vi "3.7.4-UDP-Forbrain_to_OCU-Server.vi"() -> ()   [LabVIEW 2010]
doc: "Creates a named service and listens on the first available port. Whenever a client connects to the service, it responds with a message containing joystick data. The VI can be stopped using the STOP button."
uses:
  6-OCU Neurons/CommonIndicators.ctl
  5.0-Global.vi
panel:
  out "5.7.2 Main Indicators":T1={"Speed"=0.0, " Heading"={0.0, 34.390870865624734}, "MissionTime"=0.0, "Battery"=0.0, "MAP"=FALSE, "LIDAR"=FALSE, "ManualMissionMap"=bytes[0], "ManualModeLIDAR"=bytes[0], "ManualModeStop"=FALSE, "How? 2"=FALSE, "Where? 2"=FALSE, "MWhat?"=FALSE, "ActManual"=FALSE, "CollisionLight"=FALSE, "CollisionLight 2"=FALSE, "Ready"=FALSE} {"Battery" scale=16.0..24.0; "MissionTime" scale=0.0..10.0; "Heading" scale=180.0..-180.0; "Speed" scale=0.0..4.0}
  out "data out":string
  out "error out":errorcluster
  in  "error in":errorcluster
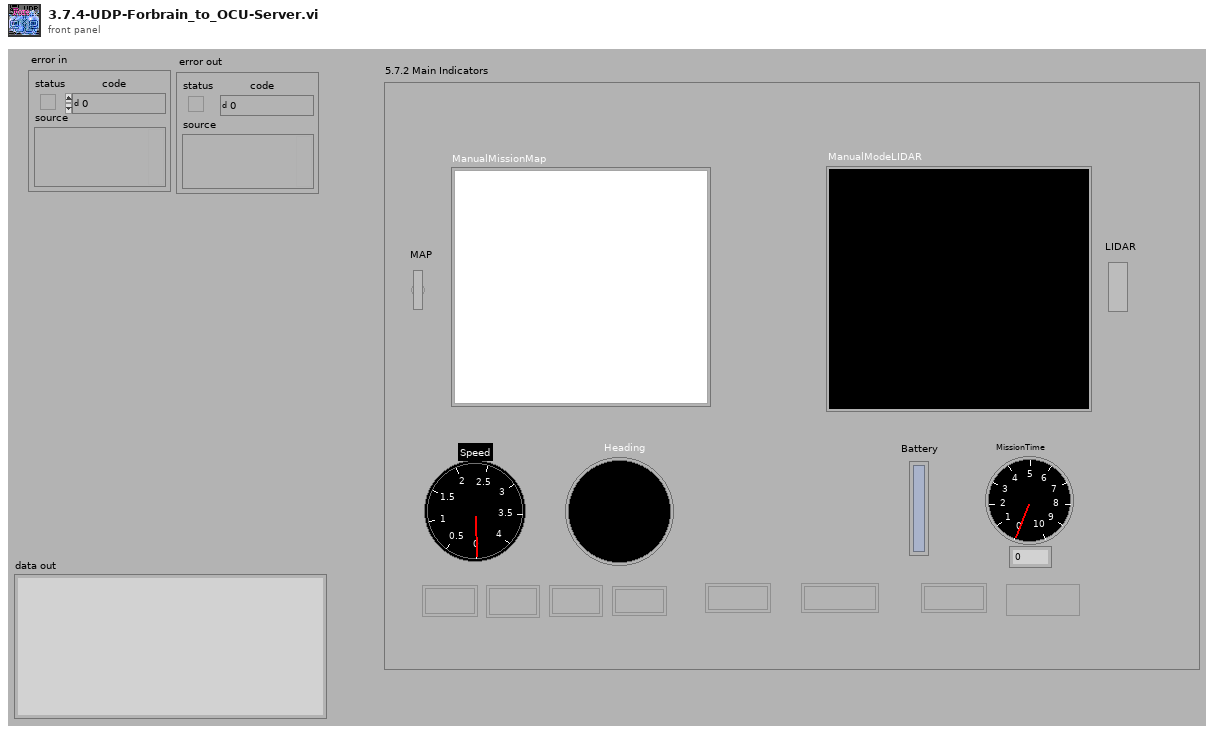
[diagram p1: front panel]
types:
  T1 = typedef "CommonIndicators.ctl" = cluster{"Speed":dbl, " Heading":cluster{dbl, dbl}, "MissionTime":dbl, "Battery":dbl, "MAP":bool, "LIDAR":bool, "ManualMissionMap":picture, "ManualModeLIDAR":picture, "ManualModeStop":bool, "How? 2":bool, "Where? 2":bool, "MWhat?":bool, "ActManual":bool, "CollisionLight":bool, "CollisionLight 2":bool, "Ready":bool}
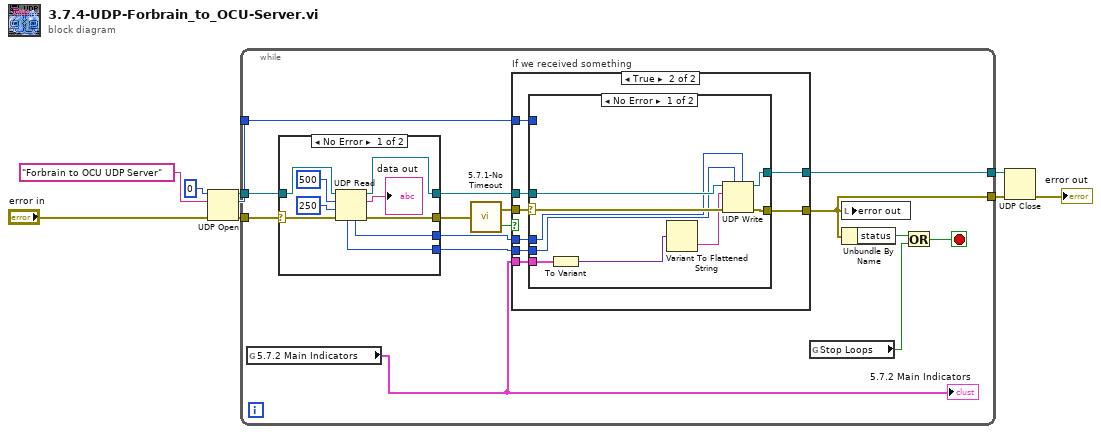
[diagram p0: block diagram]
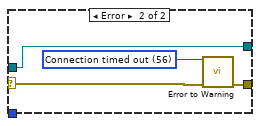
[diagram p3: hidden frame]
diagram:
  n1 = UDP Open(8:"error in", 10:"Forbrain to OCU UDP Server", 11:0) -> (port=w7:refnum<k16>, 0:w6:errorcluster, 2:w2:u16)  [unwired: 2 in]
  n2 = while {
    tunnel: [w13] -> w4
    tunnel: w7 -> [w24]
    tunnel: w6 -> [w21]
    tunnel: [w22] -> w5
    tunnel: w2 -> [w18]
    stop <- w16 stop-if-true
    n3 = global read "5.0-Global.vi" "5.7.2 Main Indicators"() -> (w10:T1)
    "5.7.2 Main Indicators" <- w10
    n4 = case shown="No Error" w21 {
      selector: w21 -> [w54 w57]
      tunnel: w24 -> [w56 w58]
      tunnel: [w53 w58] -> w23
      tunnel: [w52 w57] -> w12
      tunnel: [w50 _] -> w19
      tunnel: [w51 _] -> w20
      frame No Error {
        n5 = UDP Read(connection ID=w56, max size (548)=500, timeout ms (25000)=250, 8:w54) -> (data out=→"data out":string, error out=w52:errorcluster, 3:w53:refnum<k16>, 4:w50:u16, 6:w51:u32)
      }
      frame Error {
      }
    }
    n6 = call "5.7.1-No Timeout.vi"("error in (no error)"=w12) -> ("No Timeout"=w14:bool, "error out"=w15:errorcluster)
    n7 = case "If we received something" shown="True" w14 {
      tunnel: w23 -> [w25 w34]
      tunnel: [w25 w33] -> w22
      tunnel: w20 -> [_ w32]
      tunnel: w19 -> [_ w31]
      tunnel: w18 -> [_ w30]
      tunnel: [w26 w29] -> w13
      tunnel: w15 -> [w26 w28]
      tunnel: w10 -> [_ w27]
      frame False {
      }
      frame True {
        n8 = case shown="No Error" w28 {
          selector: w28 -> [w43 w45]
          tunnel: w34 -> [w40 w47]
          tunnel: [w42 w44] -> w29
          tunnel: [w41 w47] -> w33
          tunnel: w32 -> [w38 _]
          tunnel: w31 -> [w39 _]
          tunnel: w30 -> [_ _]
          tunnel: w27 -> [w35 _]
          frame No Error {
            n9 = To Variant(anything=w35) -> (Variant=w37:variant)
            n10 = Variant To Flattened String(Variant=w37) -> (data string=w36:string)  [unwired: 1 out]
            n11 = UDP Write(address=w38, port or service name=w39, connection ID=w40, data in=w36, 8:w43) -> (error out=w42:errorcluster, 3:w41:refnum<k16>)  [unwired: 1 in]
          }
          frame Error {
            w46 = 56 items=["No Error", "Argument Error", "Memory Full", "Out of Zone", "End of File", "File Already Open", "Generic File IO Error", "File Not Found", "File Permission Error", "Disk Full", "Duplicate Path", "Too Many Files Open", "Not Enabled", "Resource File Not Found", "Cannot Add Resource", "Resource Not Found", "Image Not Found", "Image Memory Error", "Pen Does Not Exist", "Config Bad Type", "Config Token Not Found", "Config Parse Error", "Config Memory Error", "Bad External Code Format", "Bad External Code Offset", "External Code Not Present", "Null Window", "Destroy Window Mixup", "Null Menu", "Print Aborted", "Bad Print Record", "Print Driver Error", "Windows Error During Print", "Memory Error During Print", "Print Dialog Error", "Generic Print Error", "Invalid Device Refnum", "Device Not Found", "Device Parameter Error", "Device Unit Error", "Can't Open Device", "Device Call Aborted", "Generic Error", "Cancelled By User", "Object ID Too Low", "Object ID Too High", "Object Not In Heap", "Unknown Heap", "Bad DefProc ID", "DefProc Not In Table", "Message Out Of Range", "Null Method", "Unknown Message", "Manager Call Not Supported", "Bad address", "Connection In progress", "Connection timed out", "Connection is already in progress", "Network attribute not supported", "Network error", "Address in use", "System out of memory", "Connection aborted", "Connection refused", "Connection is not connected", "Connection is already connected", "Connection closed", "Initialize error (interapplication manager)", "Bad occurrence", "Wait on unbound occurrence handler", "Occurrence queue overflow", "Bad path", "Semaphore not signaled", "Unrecognized type (interapplication manager)"] ("1st Error to Convert")
            n12 = call <vilib>:"Error to Warning.vi"("1st Error to Convert"=w46, "error in"=w45) -> ("warning out"=w44:errorcluster)  [unwired: 13 in]
          }
        }
      }
    }
    n13 = global read "5.0-Global.vi" "Stop Loops"() -> (w11:bool)
    n14 = local write "error out"(w13) -> ()
    n15 = Unbundle By Name(w13) -> ("status"=w17:bool)
    n16 = Or(x=w17, y=w11) -> (x .or. y?=w16:bool)
  }
  n17 = UDP Close(connection ID=w5, 8:w4) -> (error out=→"error out":errorcluster)  [unwired: 1 out]
